vi "plotEllipse.vi"(7 "nPoints":i32, 8 "Yradius":dbl, 9 "Ycentre":dbl, 10 "Xradius":dbl, 11 "Xcentre":dbl) -> (1 "Yarray":dbl[](array[numeric]), 2 "Xarray":dbl[](array[numeric]), 4 "plottable":cluster{"Array":dbl[], "Array":dbl[]})   [LabVIEW 2022 SP3]
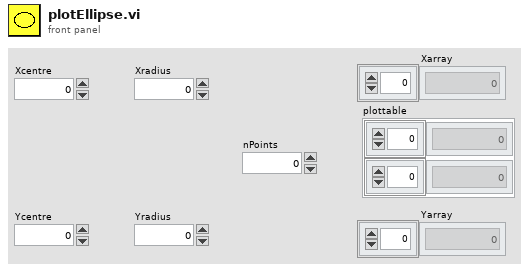
[diagram p1: front panel]
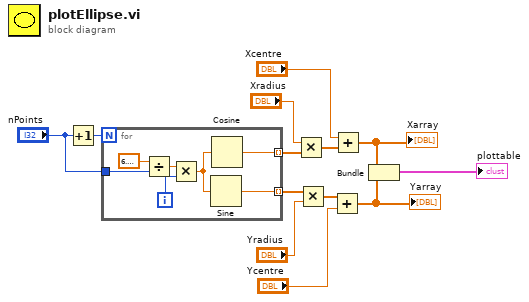
[diagram p0: block diagram]
diagram:
  n1 = Increment(x="nPoints") -> (x+1=w8:i32)
  n2 = for {
    N: w8 -> [_]
    tunnel: "nPoints" -> [w16]
    tunnel: [w15] -> w10 mode=indexing
    tunnel: [w14] -> w12 mode=indexing
    i -> [w18]
    n3 = Divide(x=6.283185307179586, y=w16) -> (x/y=w19:dbl)
    n4 = Multiply(x=w19, y=w18) -> (x*y=w17:dbl)
    n5 = Sine(x=w17) -> (sin(x)=w14:dbl)
    n6 = Cosine(x=w17) -> (cos(x)=w15:dbl)
  }
  n7 = Multiply(x="Xradius", y=w10) -> (x*y=w11:dbl[])
  n8 = Multiply(x=w12, y="Yradius") -> (x*y=w13:dbl[])
  n9 = Add(x=w13, y="Ycentre") -> (x+y=w5:dbl[])
  "Yarray" <- w5
  n10 = Add(x="Xcentre", y=w11) -> (x+y=w3:dbl[])
  "Xarray" <- w3
  n11 = Bundle(w3, w5) -> (→"plottable":cluster{dbl[], dbl[]})  [unwired: 1 in]
